vi "dfd_Error Cluster From Error Code.vi"   [LabVIEW 2017, in "NI_DigFilterLicensed.lvlib"]
uses:
  <vilib>/addons/Digital Filter Design/NI_DigFilterLicensed.lvlib
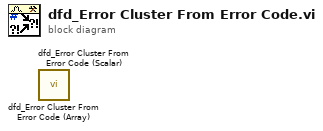
[diagram p0: block diagram]
diagram:
  n1 = call <vilib>:"dfd_Error Cluster From Error Code (Array).vi"() -> ()  [unwired: 11 in, 1 out]
  n2 = call <vilib>:"dfd_Error Cluster From Error Code (Scalar).vi"() -> ()  [unwired: 11 in, 1 out]
